vi "ep_Phase Difference Calculation.vi"(8 "error in (no error)":errorcluster, 10 "lead/lag ? (T)":bool[](array[boolean]), 11 "power values in":T1[](array[typedef])) -> (0 "error out":errorcluster, 2 "phase difference [deg]":dbl[](array[numeric]), 3 "power values out":T1[](array[typedef]))   [LabVIEW 2024]
doc: "Signs the reactive power and calculates the phase difference of input voltage and current signals."
uses:
  <vilib>/addons/Electrical Power/Basic/Measurement/subVIs/basic_Power Value.ctl
  <vilib>/addons/Electrical Power/Basic/NI_EP_Basic.lvlib
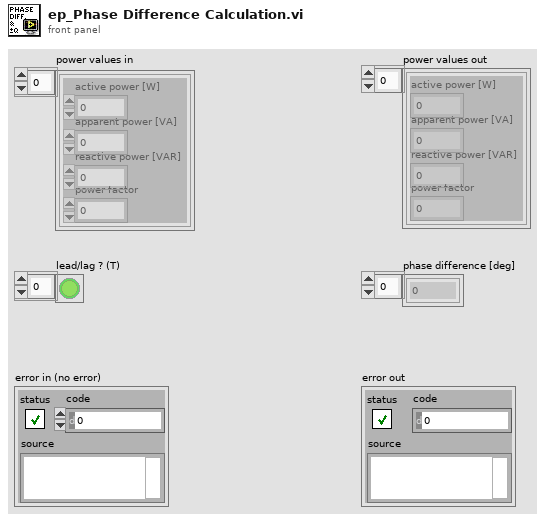
[diagram p1: front panel]
types:
  T1 = typedef "NI_EP_Basic.lvlib/basic_Power Value.ctl" = cluster{"active power [W]":dbl, "apparent power [VA]":dbl, "reactive power [VAR]":dbl, "power factor":dbl}
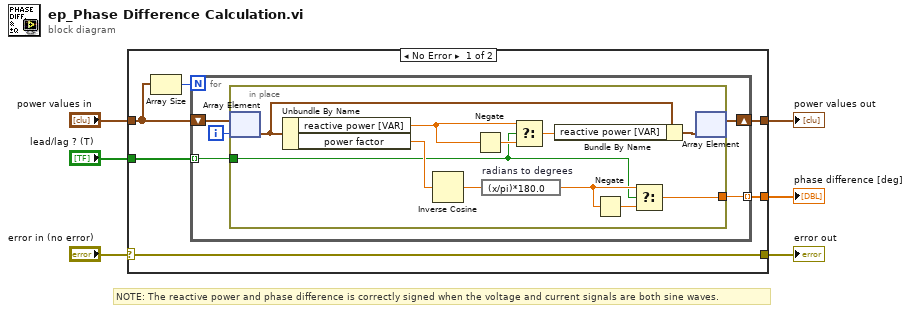
[diagram p0: block diagram]
diagram:
  # "NOTE: The reactive power and phase difference is correctly signed when the voltage and current signals are both sine waves."
  n1 = case shown="No Error" "error in (no error)" {
    selector: "error in (no error)" -> [w12 w29]
    tunnel: "power values in" -> [w9 _]
    tunnel: [w12 w29] -> w4
    tunnel: [w11 _] -> w3
    tunnel: "lead/lag ? (T)" -> [w8 _]
    tunnel: [w7 _] -> w1
    frame No Error {
      n2 = Array Size(array=w9) -> (size(s)=w10:i32)
      n3 = for {
        N: w10 -> [_]
        shift-right: [w15] -> w11
        shift-left: w9 -> [w17]
        tunnel: w8 -> [w14] mode=indexing
        tunnel: [w13] -> w7 mode=indexing
        i -> [w16]
        n4 = in-place {
          in-place-border: w14 -> [w18]
          in-place-border: [w22] -> w13
          n5 = in-place-array #1(w17, w16) -> (w25:T1)
          n6 = Unbundle By Name(w25) -> ("reactive power [VAR]"=w26:dbl, "power factor"=w23:dbl)
          n7 = Inverse Cosine(1:w23) -> (0:w19:dbl)
          n8 = Negate(x=w26) -> (-x=w27:dbl)
          n9 = expression code="(x/pi)*180.0" "radians to degrees"(w19) -> (w20:dbl)
          n10 = Select(t=w26, s=w18, f=w27) -> (s? t:f=w28:dbl)
          n11 = Bundle By Name(cluster=w25, "reactive power [VAR]"=w28) -> (w24:T1)
          n12 = Negate(x=w20) -> (-x=w21:dbl)
          n13 = Select(t=w20, s=w18, f=w21) -> (s? t:f=w22:dbl)
          n14 = in-place-array #1(w24) -> (w15:T1[])  [unwired: 1 out]
        }
      }
    }
    frame Error {
    }
  }
  "error out" <- w4
  "power values out" <- w3
  "phase difference [deg]" <- w1
